vi "Write PDF File and position [ ].vi"(8 "error in (no error)":errorcluster, 10 "PDF File and position [ ]":T1[](array[typedef]), 11 "PDF Report Class in":refnum<class "PDF Report Class.lvclass">) -> (0 "error out":errorcluster, 3 "PDF Report Class out":refnum<class "PDF Report Class.lvclass">)   [LabVIEW 2019, in "PDF Report Class.lvclass"]
uses:
  <userlib>/Exaprom PDF/LV Class/PDF Report Class/PDF Report Class.lvclass
  <userlib>/Exaprom PDF/Controls/Concatenate Controls/PDF File and position.ctl
  <userlib>/Exaprom PDF/Controls/Concatenate Controls/PDF file source.ctl
  <userlib>/Exaprom PDF/LV Class/PDF Report Class/PDF Report Class.lvclass/PDF Report Class.ctl
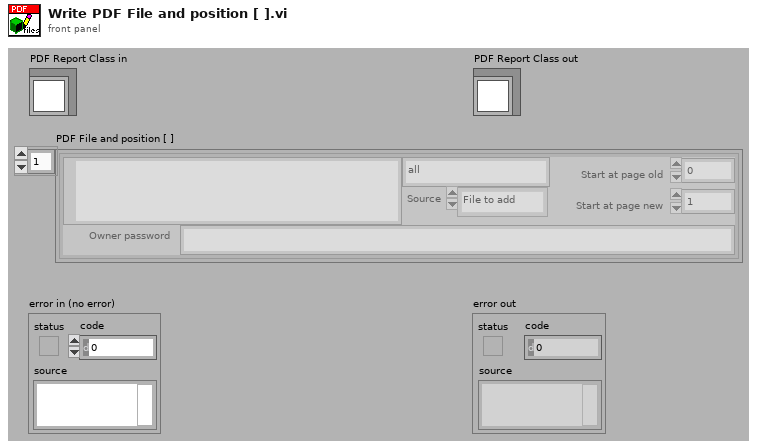
[diagram p1: front panel]
types:
  T1 = typedef "PDF File and position.ctl" = cluster{"Path":path, "Pages":string, "Source":T2, "Start at page old":i32, "Start at page new":i32, "Owner password":string}
  T2 = typedef "PDF file source.ctl" = enum16{"PDF Report", "File to add"}
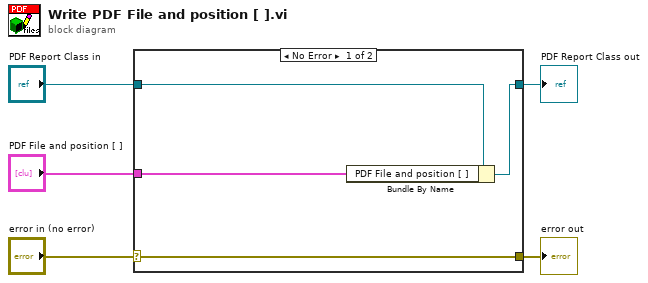
[diagram p0: block diagram]
diagram:
  n1 = case shown="No Error" "error in (no error)" {
    selector: "error in (no error)" -> [w9 w10]
    tunnel: [w9 w10] -> w4
    tunnel: [w7 w11] -> w2
    tunnel: "PDF Report Class in" -> [w8 w11]
    tunnel: "PDF File and position [ ]" -> [w6 _]
    frame No Error {
      n2 = Bundle By Name(cluster=w8, "PDF File and position [ ]"=w6) -> (w7:refnum<class "PDF Report Class.lvclass">)
    }
    frame Error {
    }
  }
  "error out" <- w4
  "PDF Report Class out" <- w2
